vi "18-tcoupl_sense_bis.vi"(3 "this":i32, 4 "unit in":i32, 5 "button":i32, 6 "settings in":T1={"Auto1"=TRUE, "Auto2"=TRUE, "Rel1"=TRUE, "Rel2"=TRUE, "Filt1"=TRUE, "Filt2"=TRUE, "Rate"=enum."Slow", "Range1"=enum."10mV", "Range2"=enum."100mV", "Filt3"=TRUE, "Filt4"=TRUE, "Rel temp 1"=TRUE, "Analog1"=FALSE, "Analog2"=FALSE, "Analog temp 1"=FALSE, "Digital1"=TRUE, "Digital2"=TRUE, "Digital temp 1 "=TRUE, "Window1"=enum."0,01%", "Window2"=enum."0,01%", "Window temp 1"=enum."0,01%", "RDGS1"="010", "RDGS2"="010", "RDGS temp 1"="010", "Type_type1"=TRUE, "Type_type2"=TRUE, "Type_type temp 1"=TRUE, "LSync"=FALSE, "Unit"=enum."C", "Sens"=TRUE, "Type tcoupl"=enum."J", "Junc"=TRUE, "prevState"=0, "Rel temp 2"=TRUE, "Analog temp 2"=FALSE, "Digital temp 2"=TRUE, "Type_type temp 2"=TRUE, "RDGS temp 2"="010", "Window temp 2"=enum."0,01%", "addres"=0}) -> (0 "next state":i32, 1 "unit out":i32, 2 "settings out":T1)   [LabVIEW 2017]
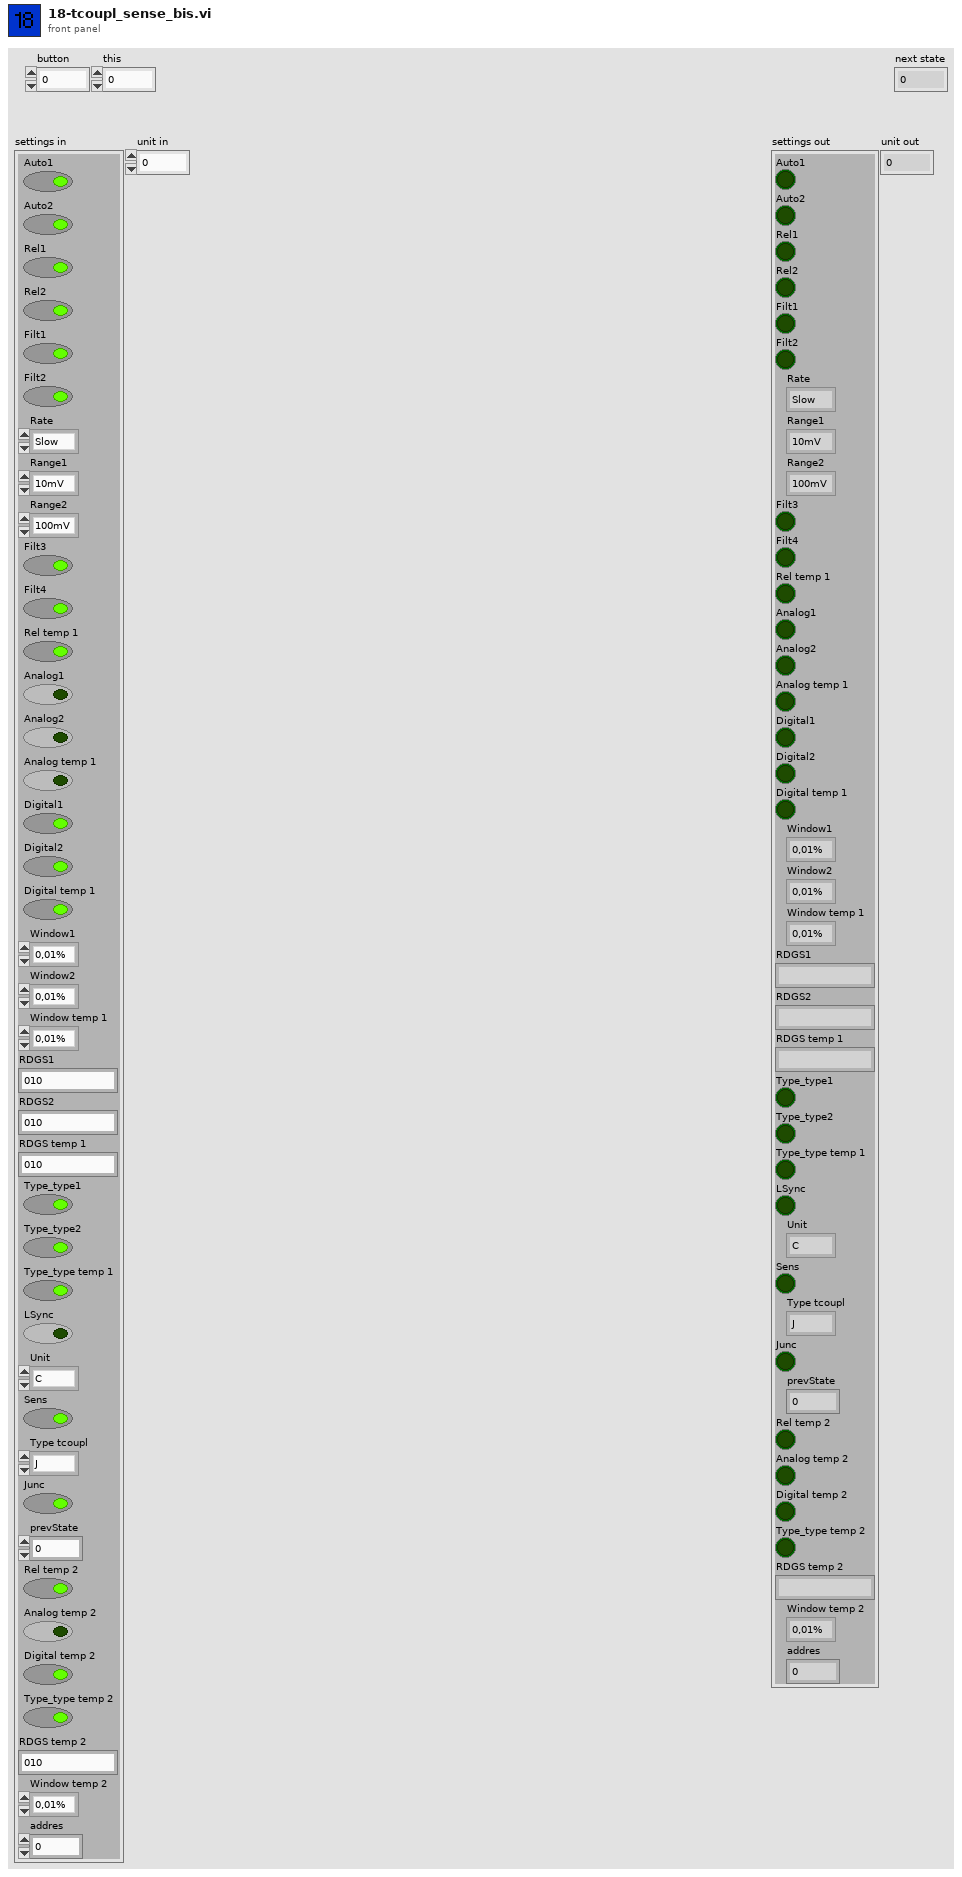
[diagram p1: front panel]
types:
  T1 = cluster{"Auto1":bool, "Auto2":bool, "Rel1":bool, "Rel2":bool, "Filt1":bool, "Filt2":bool, "Rate":enum16{"Slow", "Med", "Fast"}, "Range1":enum16{"10mV", "100mV", "1V", "10V", "100V"}, "Range2":enum16{"100mV", "1V", "10V"}, "Filt3":bool, "Filt4":bool, "Rel temp 1":bool, "Analog1":bool, "Analog2":bool, "Analog temp 1":bool, "Digital1":bool, "Digital2":bool, "Digital temp 1 ":bool, "Window1":enum16{"0,01%", "0,1%", "1%", "10%", "None"}, "Window2":enum16{"0,01%", "0,1%", "1%", "10%", "None"}, "Window temp 1":enum16{"0,01%", "0,1%", "1%", "10%", "None"}, "RDGS1":string, "RDGS2":string, "RDGS temp 1":string, "Type_type1":bool, "Type_type2":bool, "Type_type temp 1":bool, "LSync":bool, "Unit":enum16{"C", "K", "F"}, "Sens":bool, "Type tcoupl":enum16{"J", "K", "T", "E", "R", "S", "B", "N"}, "Junc":bool, "prevState":i32, "Rel temp 2":bool, "Analog temp 2":bool, "Digital temp 2":bool, "Type_type temp 2":bool, "RDGS temp 2":string, "Window temp 2":enum16{"0,01%", "0,1%", "1%", "10%", "None"}, "addres":i32}
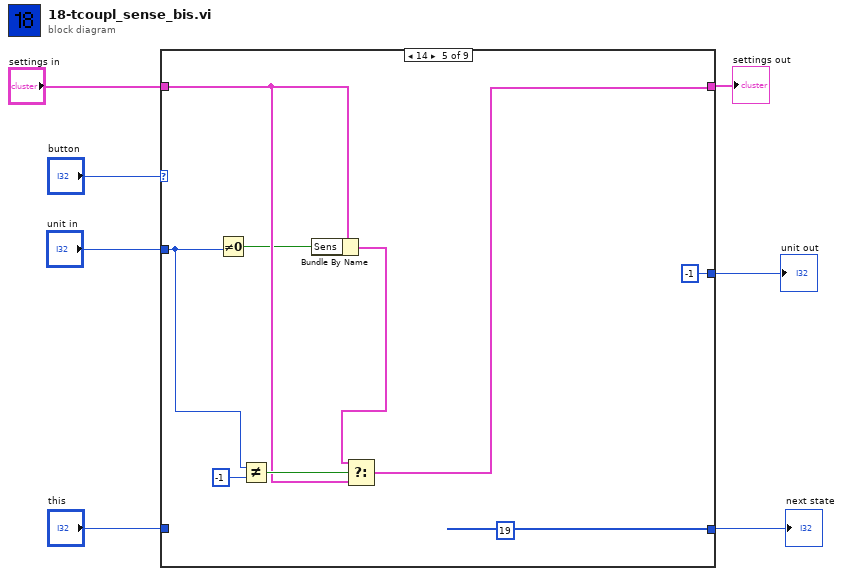
[diagram p0: block diagram]
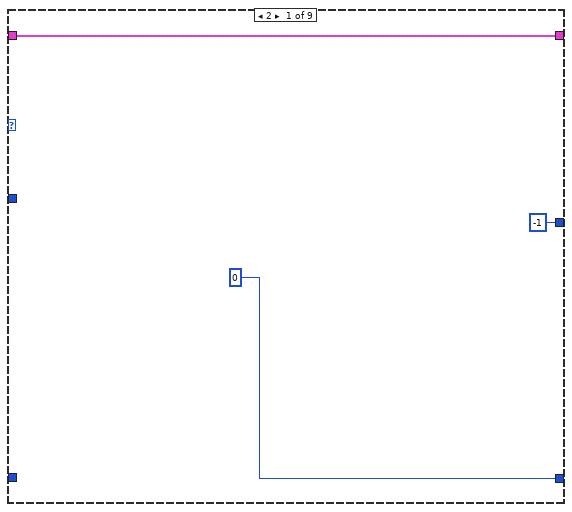
[diagram p2: hidden frame]
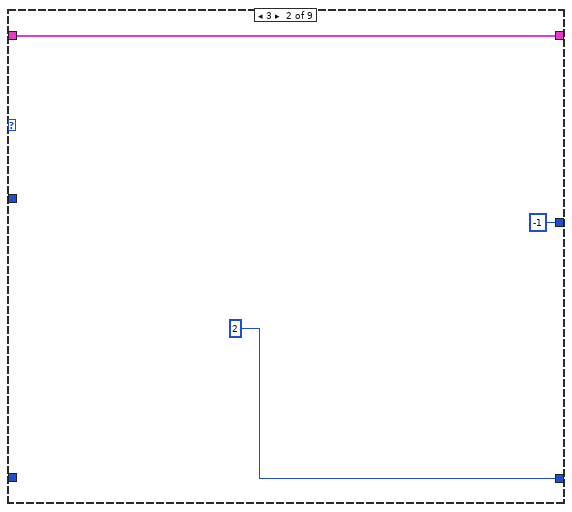
[diagram p3: hidden frame]
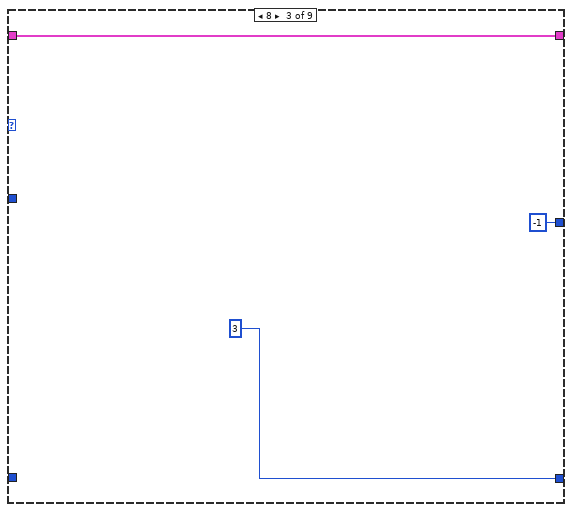
[diagram p4: hidden frame]
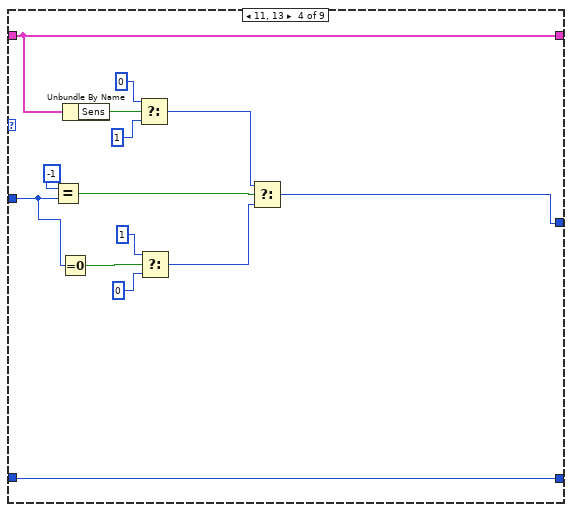
[diagram p5: hidden frame]
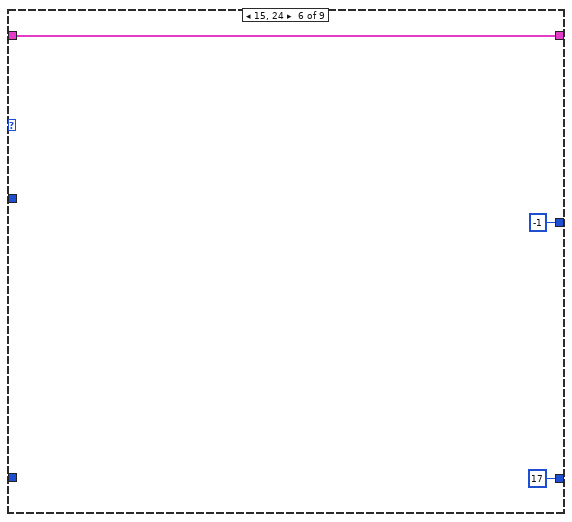
[diagram p6: hidden frame]
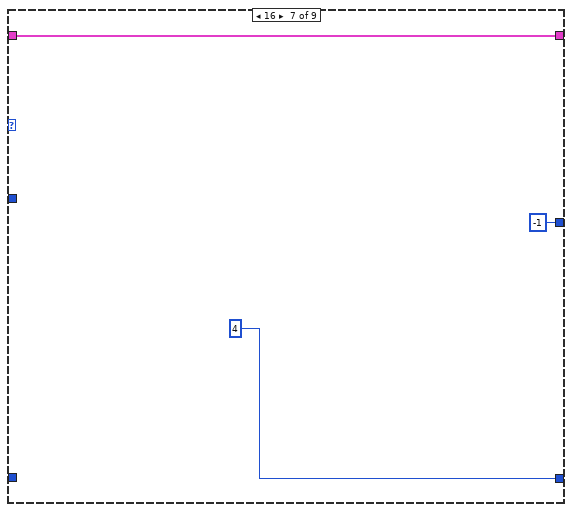
[diagram p7: hidden frame]
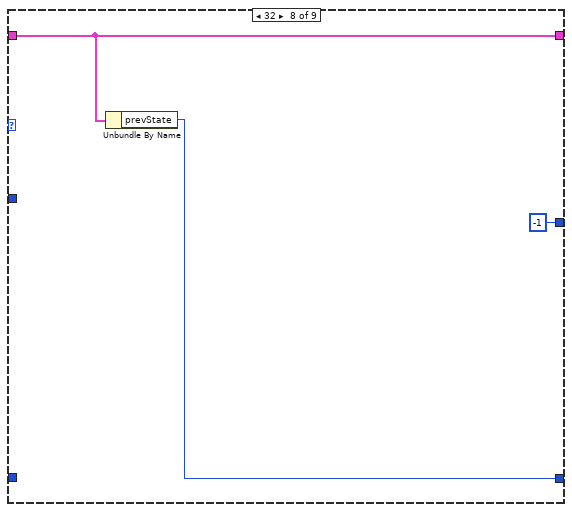
[diagram p8: hidden frame]
diagram:
  n1 = case shown="14" "button" {
    tunnel: [0 ("this") 2 3 w30 19 ("this") 17 ("prevState") 4 w47 w50] -> w5
    tunnel: "this" -> [_ _ _ w30 _ _ _ _ w50]
    tunnel: "settings in" -> [w10 w12 w15 w29 w36 w42 w44 w48 w51]
    tunnel: [w10 w12 w15 w29 w34 w42 w44 w48 w51] -> w3
    tunnel: "unit in" -> [_ _ _ w26 w32 _ _ _ w49]
    tunnel: [-1 ("window in") -1 ("window in") -1 ("window in") w17 -1 ("window in") -1 ("window in") -1 ("window in") -1 ("window in") w49] -> w1
    frame 2 {
    }
    frame 3 {
    }
    frame 8 {
    }
    frame 11, 13 {
      n2 = Equal?(x=-1, y=w26) -> (x = y?=w20:bool)
      n3 = Equal To 0?(x=w26) -> (x = 0?=w27:bool)
      n4 = Unbundle By Name(w29) -> ("Sens"=w21:bool)
      n5 = Select(t=0 ("y"), s=w21, f=1) -> (s? t:f=w19:i32)
      n6 = Select(t=1 ("y"), s=w27, f=0) -> (s? t:f=w18:i32)
      n7 = Select(t=w19, s=w20, f=w18) -> (s? t:f=w17:i32)
    }
    frame 14 {
      n8 = Not Equal To 0?(x=w32) -> (x != 0?=w31:bool)
      n9 = Not Equal?(x=w32, y=-1) -> (x != y?=w37:bool)
      n10 = Bundle By Name(cluster=w36, "Sens"=w31) -> (w35:T1)
      n11 = Select(t=w35, s=w37, f=w36) -> (s? t:f=w34:T1)
    }
    frame 15, 24 {
    }
    frame 16 {
    }
    frame 32 {
      n12 = Unbundle By Name(w48) -> ("prevState"=w47:i32)
    }
    frame Default {
    }
  }
  "next state" <- w5
  "settings out" <- w3
  "unit out" <- w1
